vi "think_and_act.vi"(8 "error in (no error)":errorcluster, 9 "antState":T1, 10 "pieceOfWorld":T4[][](array[typedef]), 11 "Igor in":refnum<class "PolyVIEW.lvclass">) -> (0 "error out":errorcluster, 2 "action":T2, 3 "Igor out":refnum<class "PolyVIEW.lvclass">)   [LabVIEW 2015, in "PolyVIEW.lvclass"]
doc: "Ant thinks and chooses action\nCreated by Artem Shevelev\nshevelev.pro\nartem@shevelev.pro\nLabVIEW Portal: https://labviewportal.org/memberlist.php?mode=viewprofile&u=2340"
uses:
  PolyVIEW.lvclass
  actors/world/typedefs/worldCell_cluster.ctl
  actors/world/typedefs/markValue_cluster.ctl
  actors/world/typedefs/markValue.ctl
  actors/world/typedefs/markVolume.ctl
  actors/world/typedefs/amountOfFood.ctl
  actors/world/typedefs/anthillType_enum.ctl
  ant_base/action_cluster.ctl
  ant_base/actionType_enum.ctl
  ant_base/antState_cluster.ctl
  ant_base/ant_base.lvclass/ant_base.ctl
  Admin memo.ctl
  ant_base/memory_limit_const.vi
  move_forvard.vi
  move_back.vi
  ant_base/ant_base.lvclass
  actors/world/world.lvlib
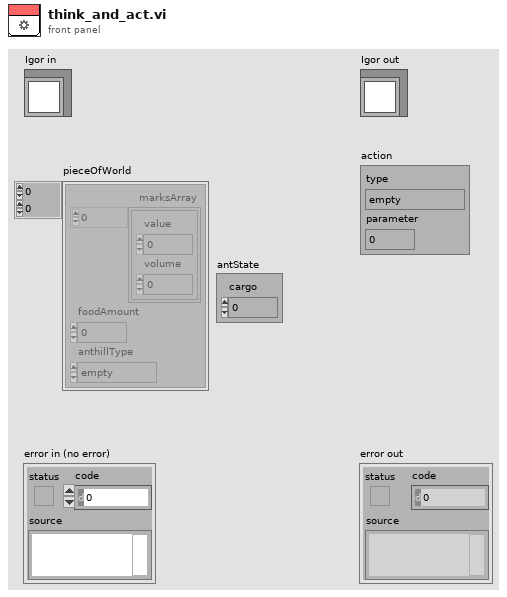
[diagram p1: front panel]
types:
  T1 = typedef "ant_base.lvclass/antState_cluster.ctl" = cluster{"cargo":u8}
  T2 = typedef "ant_base.lvclass/action_cluster.ctl" = cluster{"type":T3, "parameter":dbl}
  T3 = typedef "ant_base.lvclass/actionType_enum.ctl" = enum8{"empty", "move", "take", "put", "mark"}
  T4 = typedef "world.lvlib/worldCell_cluster.ctl" = cluster{"marksArray":T5[], "foodAmount":T8, "anthillType":T9}
  T5 = typedef "world.lvlib/markValue_cluster.ctl" = cluster{"value":T6, "volume":T7}
  T6 = typedef "world.lvlib/markValue.ctl" = u8
  T7 = typedef "world.lvlib/markVolume.ctl" = u16
  T8 = typedef "world.lvlib/amountOfFood.ctl" = i32
  T9 = typedef "world.lvlib/anthillType_enum.ctl" = enum16{"empty", "own", "rival"}
  T10 = typedef "PolyVIEW.lvclass/Admin memo.ctl" = cluster{"role":i32, "max vol":i32, "vol step":i32, "num of az":i32, "mode mark":i32, "arr of blk":i32[], "arr of az":i32[]}
  T11 = typedef "PolyVIEW.lvclass/Memory.ctl" = cluster{"role":i32, "az":i32, "blk az":i32, "steps I":u32, "add rad":i32, "steps II":u32, "mode mark":u32, "base az":u32, "num of az":u32, "mark 253":u32, "mode":u32, "commands":i32[]}
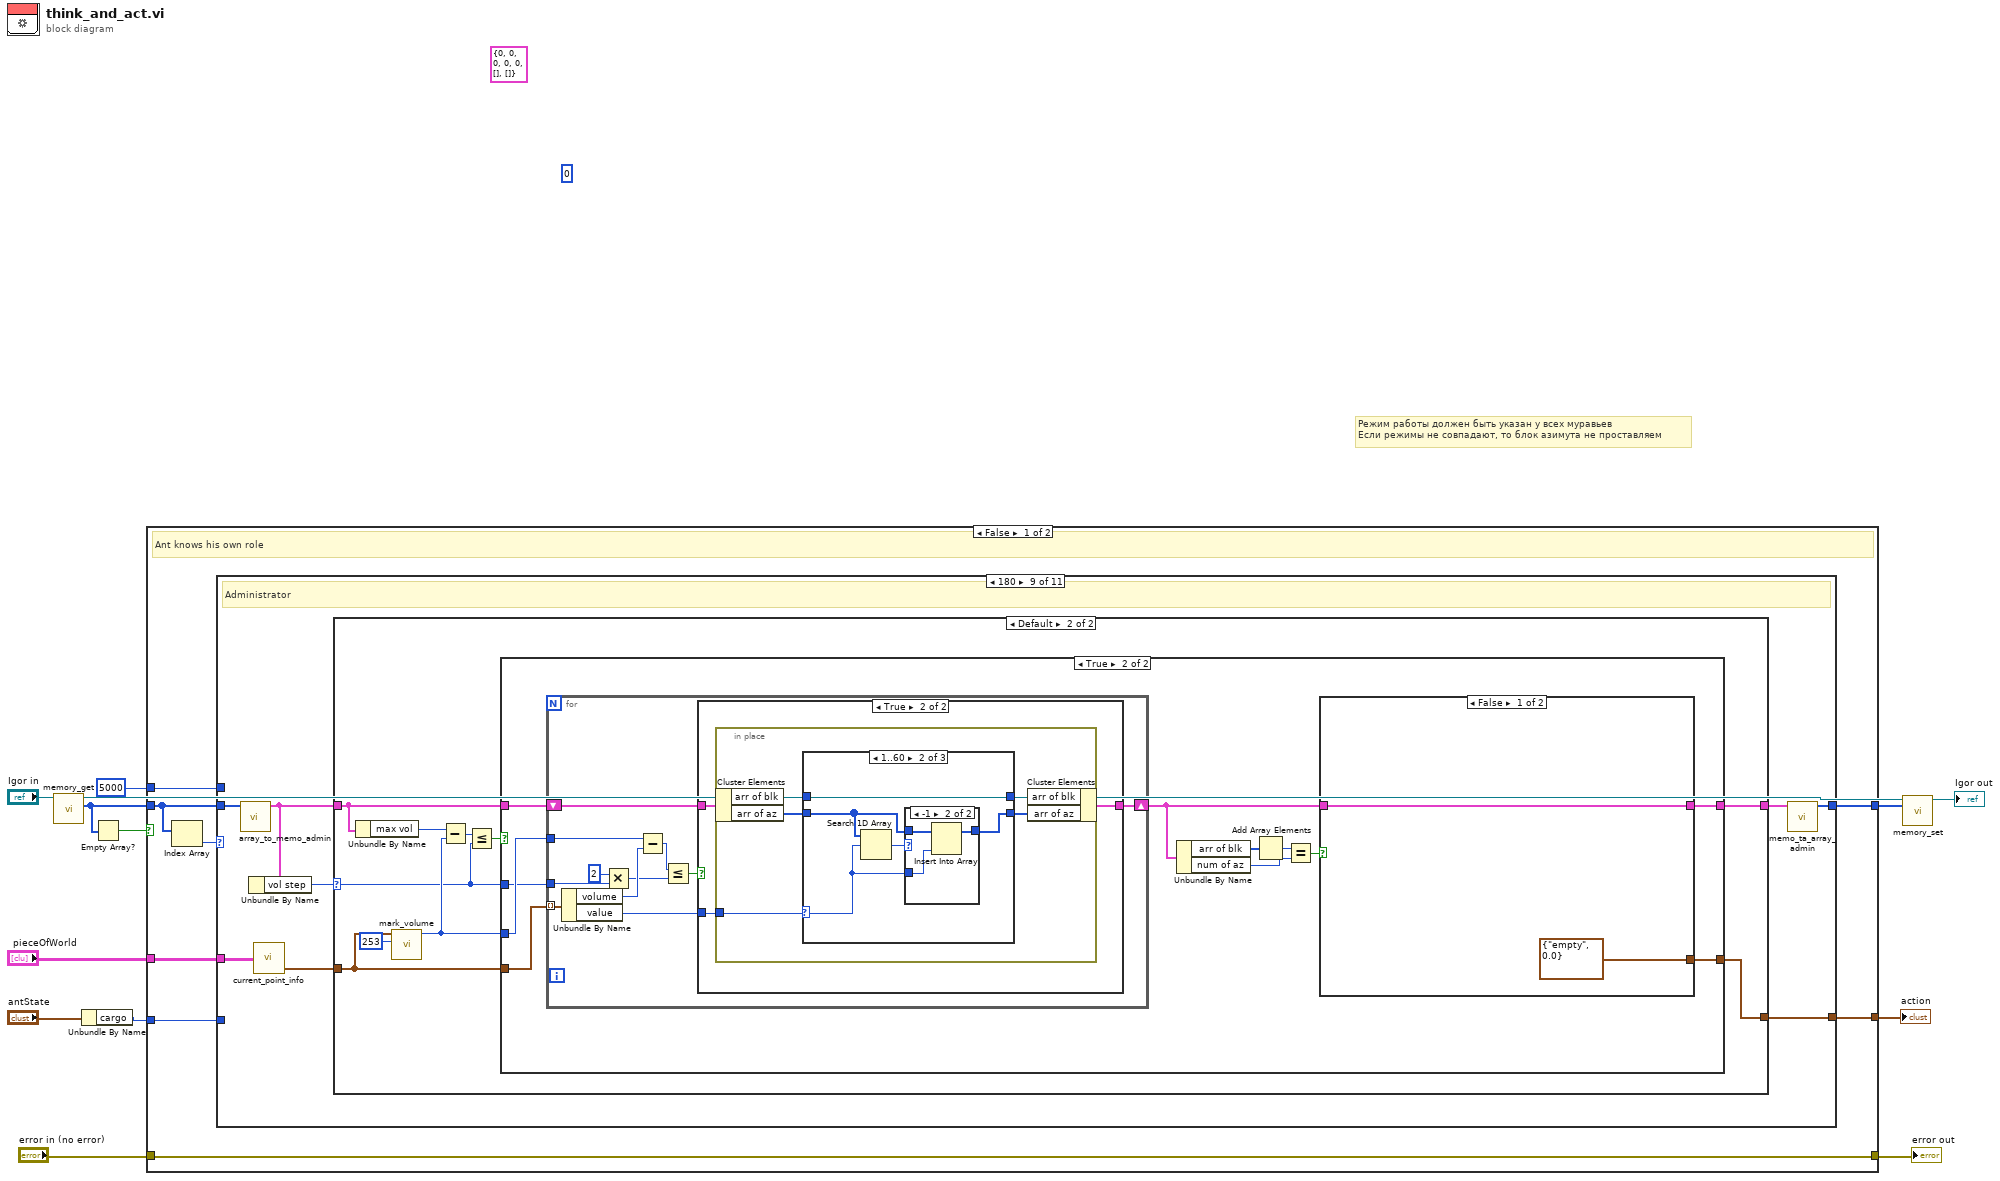
[diagram p0: block diagram]
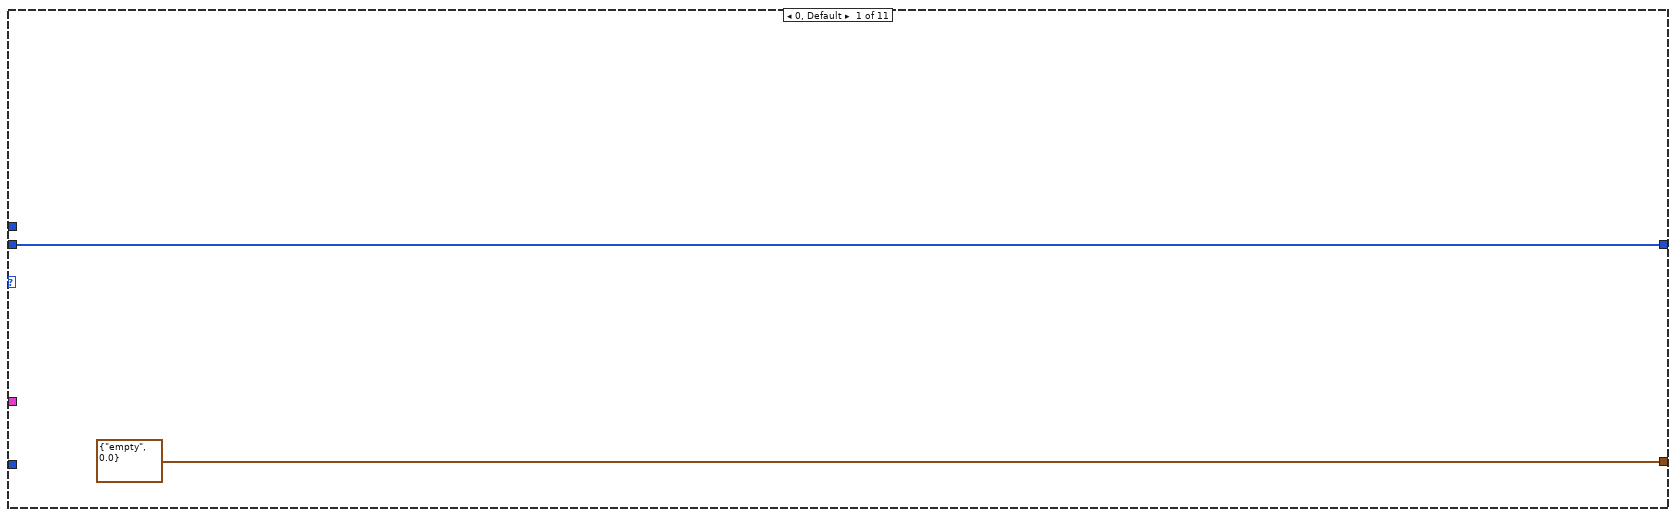
[diagram p2: hidden frame]
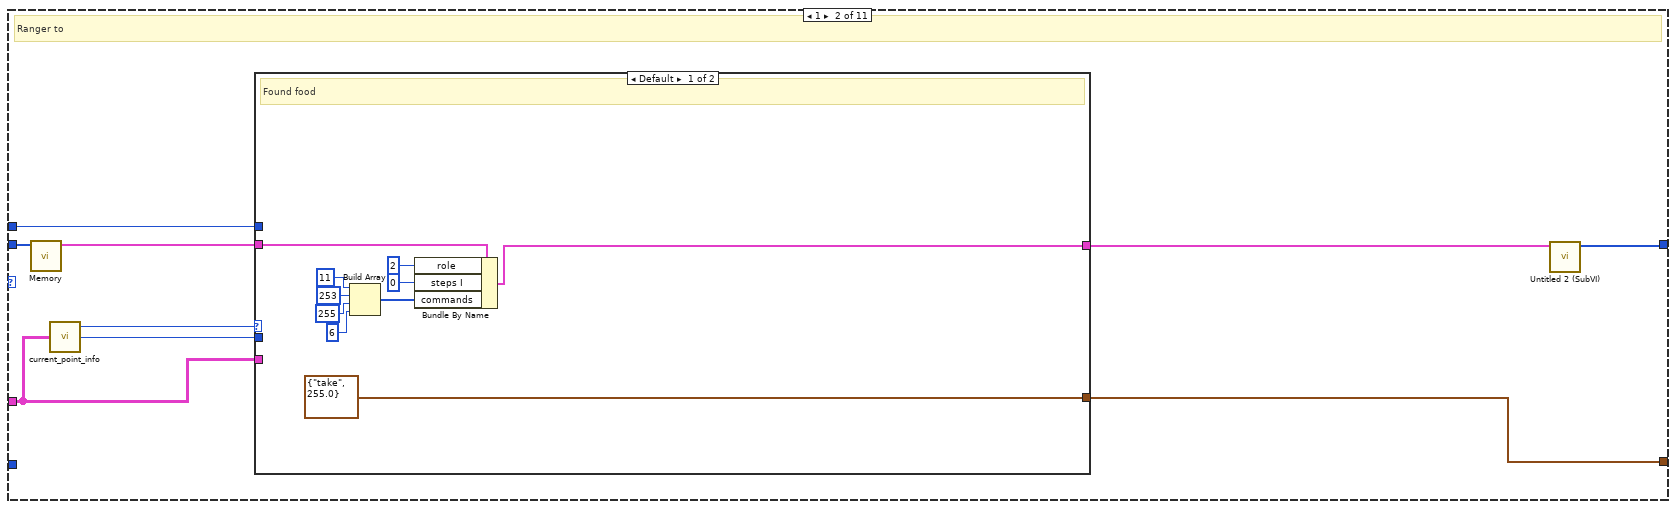
[diagram p3: hidden frame]
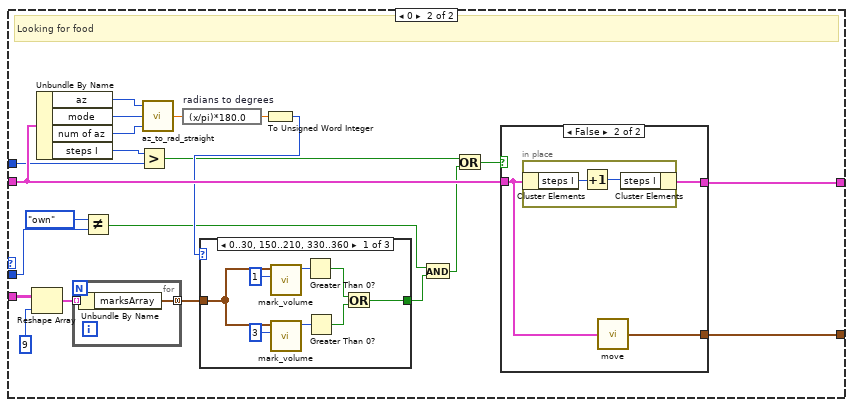
[diagram p4: hidden frame]
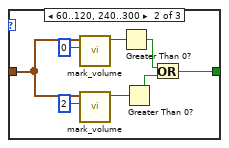
[diagram p5: hidden frame]
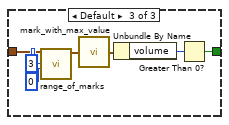
[diagram p6: hidden frame]
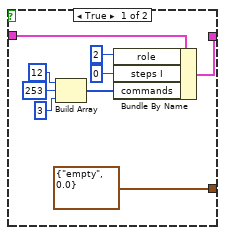
[diagram p7: hidden frame]
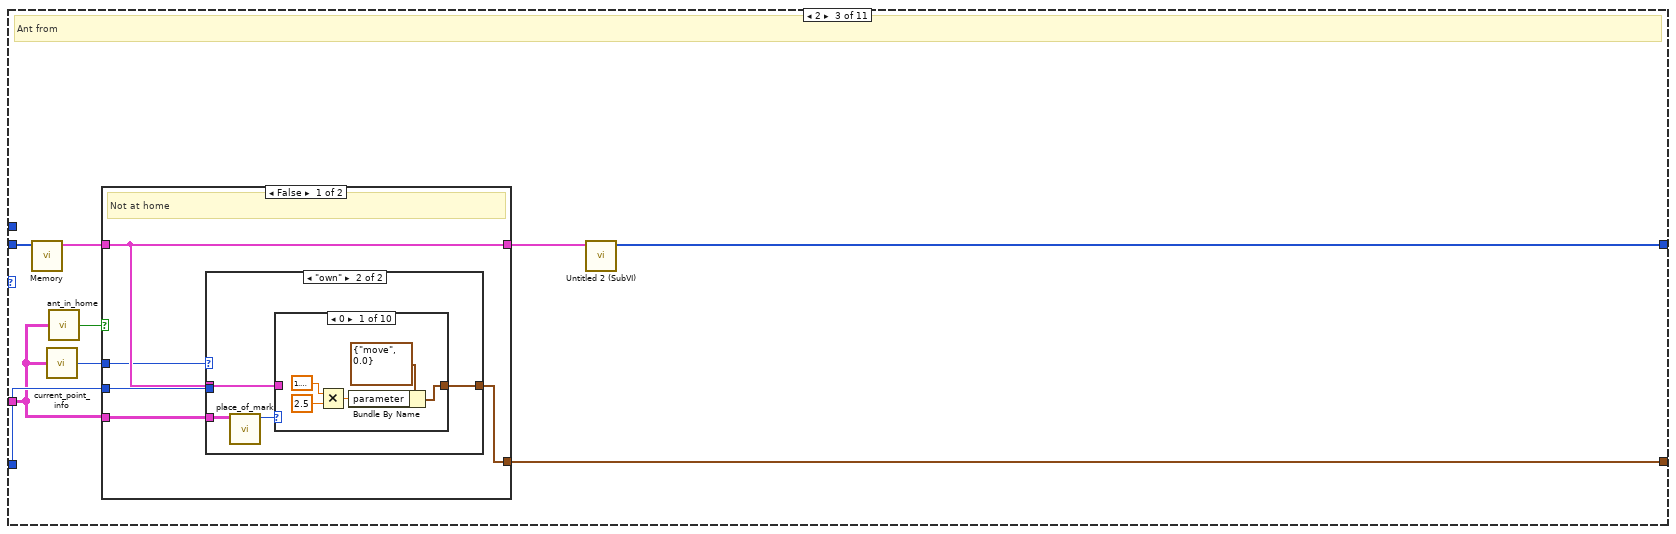
[diagram p8: hidden frame]
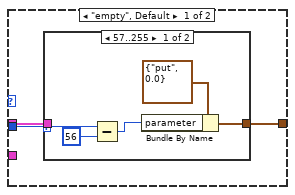
[diagram p9: hidden frame]
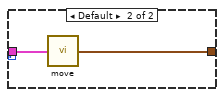
[diagram p10: hidden frame]
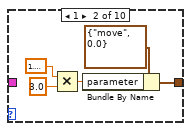
[diagram p11: hidden frame]
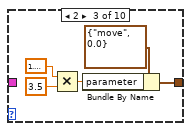
[diagram p12: hidden frame]
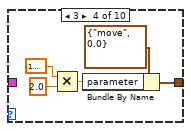
[diagram p13: hidden frame]
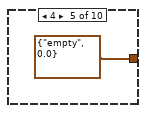
[diagram p14: hidden frame]
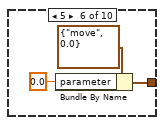
[diagram p15: hidden frame]
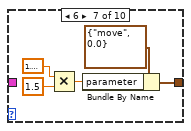
[diagram p16: hidden frame]
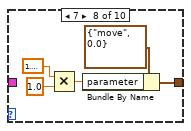
[diagram p17: hidden frame]
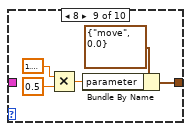
[diagram p18: hidden frame]
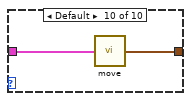
[diagram p19: hidden frame]
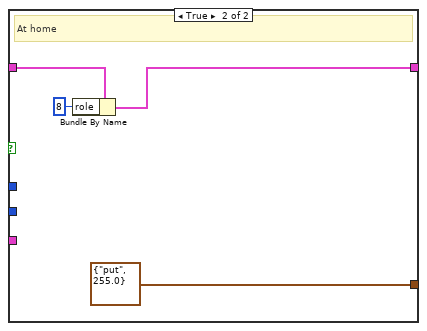
[diagram p20: hidden frame]
diagram:
  (unwired) T6 0 ("value")
  (unwired) T10 {"role"=0, "max vol"=0, "vol step"=0, "num of az"=0, "mode mark"=0, "arr of blk"=[], "arr of az"=[]}
  # "Режим работы должен быть указан у всех муравьев\nЕсли режимы не совпадают, то блок азимута не проставляем"
  n1 = call "memory_get.vi"("ant_base in"="Igor in") -> ("memory"=w3:u8[], "ant_base out"=w8:refnum<class "PolyVIEW.lvclass">)  [unwired: 8 in, 1 out]
  n2 = Unbundle By Name("antState") -> ("cargo"=w4:u8)
  n3 = Empty Array?(array=w3) -> (empty?=w10:bool)
  n4 = case shown="False" w10 {
    tunnel: [w14 w737] -> w5
    tunnel: [w20 w736] -> w13
    tunnel: "error in (no error)" -> [w14 w737]
    tunnel: w3 -> [w19 w733]
    tunnel: "pieceOfWorld" -> [w18 w732]
    tunnel: [w17 w734] -> w7
    tunnel: w4 -> [w16 _]
    tunnel: u32 5000 ("y") -> [w15 _]
    frame False {
      # "Ant knows his own role"
      n5 = Index Array(array=w19) -> (element=w21:u8)  [unwired: 1 in]
      n6 = case shown="180" w21 {
        tunnel: [T2 {"type"=enum."empty", "parameter"=0.0} ("action") w32 w112 T2 {"type"=enum."empty", "parameter"=0.0} ("action") w244 w321 w402 w462 w586 T2 {"type"=enum."mark", "parameter"=254.0} ("action") T2 {"type"=enum."empty", "parameter"=0.0} ("action")] -> w20
        tunnel: w19 -> [w22 w30 w110 w191 w242 w319 w404 w463 w583 w723 w728]
        tunnel: w18 -> [_ w31 w104 w182 w243 w320 w392 w459 w585 _ _]
        tunnel: [w22 w27 w107 w189 w239 w316 w403 w461 w579 w722 w727] -> w17
        tunnel: w16 -> [_ _ w106 _ _ _ _ _ _ _ _]
        tunnel: w15 -> [_ w26 _ _ w236 w313 _ _ _ _ _]
        frame 0, Default {
        }
        frame 1 {
          # "Ranger to"
          n7 = call "Memory.vi"("memory"=w30) -> ("output cluster"=w29:T11)  [unwired: 10 in]
          n8 = call "current_point_info.vi"("pieceOfWorld"=w31) -> ("foodAmount"=w25:T8, "anthillType"=w24:T9)  [unwired: 1 out]
          n9 = case shown="Default" w25 {
            tunnel: [T2 {"type"=enum."take", "parameter"=255.0} ("action") w64] -> w32
            tunnel: w29 -> [w40 w58]
            tunnel: [w39 w63] -> w28
            tunnel: w31 -> [_ w60]
            tunnel: w24 -> [_ w52]
            tunnel: w26 -> [_ w45]
            frame Default {
              # "Found food"
              n10 = Build Array(11 ("element"), 253 ("element"), 255 ("element"), 6 ("element")) -> (w35:i32[])
              n11 = Bundle By Name(cluster=w40, "role"=u8 2 ("new element/subarray"), "steps I"=u32 0 ("Steps I"), "commands"=w35) -> (w39:T11)
            }
            frame 0 {
              # "Looking for food"
              n12 = Reshape Array(w60, 9 ("dimension size")) -> (w61:T4[])
              n13 = Unbundle By Name(w58) -> ("az"=w43:i32, "mode"=w44:u32, "num of az"=w57:u32, "steps I"=w49:u32)
              n14 = for {
                tunnel: w61 -> [w89] mode=indexing
                tunnel: [w88] -> w59 mode=concatenating
                n15 = Unbundle By Name(w89) -> ("marksArray"=w88:T5[])
              }
              n16 = Not Equal?(x=anthillType_enum."own", y=w52) -> (x != y?=w50:bool)
              n17 = Greater?(x=w49, y=w45) -> (0:w48:bool)
              n18 = call "az_to_rad_straight.vi"("az quantity"=w57, "mode"=w44, "az"=w43) -> ("rad"=w56:dbl)
              n19 = expression code="(x/pi)*180.0" "radians to degrees"(w56) -> (w55:dbl)
              n20 = To Unsigned Word Integer(number=w55) -> (unsigned 16bit integer=w54:u16)
              n21 = case shown="0..30, 150..210, 330..360" w54 {
                tunnel: w59 -> [w72 w80 w85]
                tunnel: [w65 w73 w81] -> w53
                frame 0..30, 150..210, 330..360 {
                  n22 = call "mark_volume.vi"("element"=T6 1, "marksArray"=w72) -> ("volume"=w68:T7)  [unwired: 9 in]
                  n23 = call "mark_volume.vi"("element"=T6 3, "marksArray"=w72) -> ("volume"=w69:T7)  [unwired: 9 in]
                  n24 = Greater Than 0?(x=w68) -> (x > 0?=w66:bool)
                  n25 = Greater Than 0?(x=w69) -> (x > 0?=w67:bool)
                  n26 = Or(x=w66, y=w67) -> (x .or. y?=w65:bool)
                }
                frame 60..120, 240..300 {
                  n27 = call "mark_volume.vi"("element"=T6 0, "marksArray"=w80) -> ("volume"=w76:T7)  [unwired: 9 in]
                  n28 = call "mark_volume.vi"("element"=T6 2, "marksArray"=w80) -> ("volume"=w77:T7)  [unwired: 9 in]
                  n29 = Greater Than 0?(x=w76) -> (x > 0?=w74:bool)
                  n30 = Greater Than 0?(x=w77) -> (x > 0?=w75:bool)
                  n31 = Or(x=w74, y=w75) -> (x .or. y?=w73:bool)
                }
                frame Default {
                  n32 = call "range_of_marks.vi"("lower limit"=T6 0, "upper limit"=T6 3, "marksArray"=w85) -> ("Array"=w84:T5[])  [unwired: 8 in]
                  n33 = call "mark_with_max_value.vi"("marksArray"=w84) -> ("markValue"=w83:T5)
                  n34 = Unbundle By Name(w83) -> ("volume"=w82:T7)
                  n35 = Greater Than 0?(x=w82) -> (x > 0?=w81:bool)
                }
              }
              n36 = And(x=w50, y=w53) -> (x .and. y?=w47:bool)
              n37 = Or(x=w48, y=w47) -> (x .or. y?=w46:bool)
              n38 = case shown="False" w46 {
                tunnel: [T2 {"type"=enum."empty", "parameter"=0.0} ("action") w101] -> w64
                tunnel: w58 -> [w95 w100]
                tunnel: [w96 w99] -> w63
                frame True {
                  n39 = Build Array(12 ("element"), 253 ("element"), 3 ("element")) -> (w91:i32[])
                  n40 = Bundle By Name(cluster=w95, "role"=u8 2 ("new element/subarray"), "steps I"=u32 0 ("Steps I"), "commands"=w91) -> (w96:T11)
                }
                frame False {
                  n41 = in-place {
                    n42 = in-place-cluster #1(w100) -> ("steps I"=w103:u32)
                    n43 = Increment(x=w103) -> (x+1=w102:u32)
                    n44 = in-place-cluster #1("steps I"=w102) -> (w99:T11)
                  }
                  n45 = call-poly "move.vi"("output cluster"=w100) -> ("action"=w101:T2)
                }
              }
            }
          }
          n46 = call "Untitled 2 (SubVI).vi"(11:w28) -> ("appended array"=w27:u32[])  [unwired: 10 in]
        }
        frame 2 {
          # "Ant from"
          n47 = call "Memory.vi"("memory"=w110) -> ("output cluster"=w109:T11)  [unwired: 10 in]
          n48 = call "current_point_info.vi"("pieceOfWorld"=w104) -> ("anthillType"=w105:T9)  [unwired: 2 out]
          n49 = call "ant_in_home.vi"("pieceOfWorld"=w104) -> ("x .and. y?"=w111:bool)
          n50 = case shown="False" w111 {
            tunnel: [w116 T2 {"type"=enum."put", "parameter"=255.0} ("action")] -> w112
            tunnel: w109 -> [w117 w176]
            tunnel: [w117 w173] -> w108
            tunnel: w106 -> [w115 _]
            tunnel: w105 -> [w114 _]
            tunnel: w104 -> [w113 _]
            frame False {
              # "Not at home"
              n51 = case shown="\"own\"" w114 {
                tunnel: w117 -> [w120 w130]
                tunnel: [w119 w129] -> w116
                tunnel: w115 -> [w118 _]
                tunnel: w113 -> [_ w128]
                frame "empty", Default {
                  n52 = case shown="57..255" w118 {
                    selector: w118 -> [w124 _]
                    tunnel: w120 -> [_ w127]
                    tunnel: [w121 w126] -> w119
                    frame 57..255 {
                      n53 = Subtract(x=w124, y=u8 56) -> (x-y=w122:u8)
                      n54 = Bundle By Name(cluster=T2 {"type"=enum."put", "parameter"=0.0} ("action"), "parameter"=w122) -> (w121:T2)
                    }
                    frame Default {
                      n55 = call-poly "move.vi"("output cluster"=w127) -> ("action"=w126:T2)
                    }
                  }
                }
                frame "own" {
                  n56 = call "place_of_mark.vi"("pieceOfWorld in"=w128) -> ("f"=w131:i32)  [unwired: 10 in]
                  n57 = case shown="0" w131 {
                    tunnel: w130 -> [_ _ _ _ _ _ _ _ _ w172]
                    tunnel: [w136 w141 w146 w151 T2 {"type"=enum."empty", "parameter"=0.0} ("action") w155 w160 w165 w170 w171] -> w129
                    frame 0 {
                      n58 = Multiply(x=1.5707963267948966, y=2.5) -> (x*y=w132:dbl)
                      n59 = Bundle By Name(cluster=T2 {"type"=enum."move", "parameter"=0.0} ("action"), "parameter"=w132) -> (w136:T2)
                    }
                    frame 1 {
                      n60 = Multiply(x=1.5707963267948966, y=3.0) -> (x*y=w137:dbl)
                      n61 = Bundle By Name(cluster=T2 {"type"=enum."move", "parameter"=0.0} ("action"), "parameter"=w137) -> (w141:T2)
                    }
                    frame 2 {
                      n62 = Multiply(x=1.5707963267948966, y=3.5) -> (x*y=w142:dbl)
                      n63 = Bundle By Name(cluster=T2 {"type"=enum."move", "parameter"=0.0} ("action"), "parameter"=w142) -> (w146:T2)
                    }
                    frame 3 {
                      n64 = Multiply(x=1.5707963267948966, y=2.0) -> (x*y=w147:dbl)
                      n65 = Bundle By Name(cluster=T2 {"type"=enum."move", "parameter"=0.0} ("action"), "parameter"=w147) -> (w151:T2)
                    }
                    frame 4 {
                    }
                    frame 5 {
                      n66 = Bundle By Name(cluster=T2 {"type"=enum."move", "parameter"=0.0} ("action"), "parameter"=0.0) -> (w155:T2)
                    }
                    frame 6 {
                      n67 = Multiply(x=1.5707963267948966, y=1.5) -> (x*y=w156:dbl)
                      n68 = Bundle By Name(cluster=T2 {"type"=enum."move", "parameter"=0.0} ("action"), "parameter"=w156) -> (w160:T2)
                    }
                    frame 7 {
                      n69 = Multiply(x=1.5707963267948966, y=1.0) -> (x*y=w161:dbl)
                      n70 = Bundle By Name(cluster=T2 {"type"=enum."move", "parameter"=0.0} ("action"), "parameter"=w161) -> (w165:T2)
                    }
                    frame 8 {
                      n71 = Multiply(x=1.5707963267948966, y=0.5) -> (x*y=w166:dbl)
                      n72 = Bundle By Name(cluster=T2 {"type"=enum."move", "parameter"=0.0} ("action"), "parameter"=w166) -> (w170:T2)
                    }
                    frame Default {
                      n73 = call-poly "move.vi"("output cluster"=w172) -> ("action"=w171:T2)
                    }
                  }
                }
              }
            }
            frame True {
              # "At home"
              n74 = Bundle By Name(cluster=w176, "role"=u8 8 ("y")) -> (w173:T11)
            }
          }
          n75 = call "Untitled 2 (SubVI).vi"(11:w108) -> ("appended array"=w107:u32[])  [unwired: 10 in]
        }
        frame 3 {
          # "Ant-on-duty"
          n76 = call "Memory.vi"("memory"=w191) -> ("output cluster"=w180:T11)  [unwired: 10 in]
          n77 = call "current_point_info.vi"("pieceOfWorld"=w182) -> ("marksArray"=w179:T5[])  [unwired: 2 out]
          n78 = call "range_of_marks.vi"("lower limit"=T6 251, "upper limit"=T6 252, "marksArray"=w179) -> ("Array"=w186:T5[])  [unwired: 8 in]
          n79 = call "mark_with_max_volume.vi"("marksArray"=w186) -> ("markValue"=w185:T5)
          n80 = Unbundle By Name(w180) -> ("mode mark"=w178:u32)
          n81 = Unbundle By Name(w185) -> ("value"=w177:T6)
          n82 = Equal To 0?(x=w177) -> (x = 0?=w183:bool)
          n83 = Equal?(x=w178, y=w177) -> (x = y?=w184:bool)
          n84 = Or(x=w184, y=w183) -> (x .or. y?=w181:bool)
          n85 = case shown="True" w181 {
            tunnel: [w197 w223] -> w190
            tunnel: w180 -> [w196 w222]
            tunnel: w179 -> [_ w216]
            tunnel: w177 -> [w193 _]
            frame False {
              n86 = Unbundle By Name(w196) -> ("base az"=w194:u32, "mode"=w195:u32)
              n87 = case shown="Default" w194 {
                selector: w194 -> [w199 _]
                tunnel: [w202 w210] -> w197
                tunnel: w196 -> [w203 w209]
                tunnel: w195 -> [w201 w207]
                tunnel: w193 -> [w198 w205]
                frame Default {
                  n88 = Increment(x=w201) -> (x+1=w200:u32)
                  n89 = Bundle By Name(cluster=w203, "role"=1, "az"=w199, "mode"=w200, "mode mark"=w198) -> (w202:T11)
                }
                frame 0 {
                  n90 = Increment(x=w207) -> (x+1=w206:u32)
                  n91 = Bundle By Name(cluster=w209, "role"=3, "mode"=w206, "mode mark"=w205) -> (w210:T11)
                }
              }
            }
            frame True {
              n92 = call "range_of_marks.vi"("lower limit"=T6 121, "upper limit"=T6 180, "marksArray"=w216) -> ("Array"=w218:T5[])  [unwired: 8 in]
              n93 = call "range_of_marks.vi"("lower limit"=T6 254, "upper limit"=T6 255, "marksArray"=w216) -> ("Array"=w212:T5[])  [unwired: 8 in]
              n94 = call "mark_with_max_volume.vi"("marksArray"=w218) -> ("markValue"=w219:T5)
              n95 = call "mark_with_max_volume.vi"("marksArray"=w212) -> ("markValue"=w213:T5)
              n96 = Unbundle By Name(w219) -> ("value"=w217:T6)
              n97 = Unbundle By Name(w213) -> ("value"=w211:T6)
              n98 = case shown="255" w211 {
                tunnel: [w224 w227] -> w223
                tunnel: w222 -> [w224 w226]
                tunnel: w217 -> [_ w225]
                frame 254, Default {
                }
                frame 255 {
                  n99 = case shown="121..180" w225 {
                    selector: w225 -> [w233 _]
                    tunnel: w226 -> [w230 w235]
                    tunnel: [w234 w235] -> w227
                    frame 121..180 {
                      # "Got a target"
                      n100 = Subtract(x=w233, y=T6 120) -> (x-y=w231:T6)
                      n101 = Bundle By Name(cluster=w230, "role"=4 ("Role"), "az"=w231, "steps I"=u32 0 ("Steps I")) -> (w234:T11)
                    }
                    frame Default {
                      # "Expecting a target"
                    }
                  }
                }
              }
            }
          }
          n102 = call "Untitled 2 (SubVI).vi"(11:w190) -> ("appended array"=w189:u32[])  [unwired: 10 in]
        }
        frame 4 {
          # "Worker to"
          n103 = call "Memory.vi"("memory"=w242) -> ("output cluster"=w241:T11)  [unwired: 10 in]
          n104 = call "current_point_info.vi"("pieceOfWorld"=w243) -> ("foodAmount"=w238:T8, "anthillType"=w237:T9)  [unwired: 1 out]
          n105 = case shown="0" w238 {
            tunnel: [T2 {"type"=enum."take", "parameter"=255.0} ("action") w273] -> w244
            tunnel: w241 -> [w250 w267]
            tunnel: [w249 w272] -> w240
            tunnel: w243 -> [_ w269]
            tunnel: w237 -> [_ w259]
            tunnel: w236 -> [_ w256]
            frame Default {
              # "Found food"
              n106 = Build Array(255 ("element"), 3 ("element")) -> (w247:i32[])
              n107 = Bundle By Name(cluster=w250, "role"=u8 2 ("new element/subarray"), "steps I"=u32 0 ("Steps I"), "commands"=w247) -> (w249:T11)
            }
            frame 0 {
              # "Looking for food"
              n108 = Reshape Array(w269, 9 ("dimension size")) -> (w270:T4[])
              n109 = Unbundle By Name(w267) -> ("az"=w266:i32, "num of az"=w265:u32, "steps I"=w257:u32)
              n110 = for {
                tunnel: w270 -> [w298] mode=indexing
                tunnel: [w297] -> w268 mode=concatenating
                n111 = Unbundle By Name(w298) -> ("marksArray"=w297:T5[])
              }
              n112 = Not Equal?(x=anthillType_enum."own", y=w259) -> (x != y?=w258:bool)
              n113 = Greater?(x=w257, y=w256) -> (0:w253:bool)
              n114 = call "az_to_rad_straight.vi"("az quantity"=w265, "az"=w266) -> ("rad"=w264:dbl)  [unwired: 1 in]
              n115 = expression code="(x/pi)*180.0" "radians to degrees"(w264) -> (w263:dbl)
              n116 = To Unsigned Word Integer(number=w263) -> (unsigned 16bit integer=w262:u16)
              n117 = case shown="60..120, 240..300" w262 {
                tunnel: w268 -> [w281 w289 w294]
                tunnel: [w274 w282 w290] -> w261
                frame 0..30, 150..210, 330..360 {
                  n118 = call "mark_volume.vi"("element"=T6 1, "marksArray"=w281) -> ("volume"=w277:T7)  [unwired: 9 in]
                  n119 = call "mark_volume.vi"("element"=T6 3, "marksArray"=w281) -> ("volume"=w278:T7)  [unwired: 9 in]
                  n120 = Greater Than 0?(x=w277) -> (x > 0?=w275:bool)
                  n121 = Greater Than 0?(x=w278) -> (x > 0?=w276:bool)
                  n122 = Or(x=w275, y=w276) -> (x .or. y?=w274:bool)
                }
                frame 60..120, 240..300 {
                  n123 = call "mark_volume.vi"("element"=T6 0, "marksArray"=w289) -> ("volume"=w285:T7)  [unwired: 9 in]
                  n124 = call "mark_volume.vi"("element"=T6 2, "marksArray"=w289) -> ("volume"=w286:T7)  [unwired: 9 in]
                  n125 = Greater Than 0?(x=w285) -> (x > 0?=w283:bool)
                  n126 = Greater Than 0?(x=w286) -> (x > 0?=w284:bool)
                  n127 = Or(x=w283, y=w284) -> (x .or. y?=w282:bool)
                }
                frame Default {
                  n128 = call "range_of_marks.vi"("lower limit"=T6 0, "upper limit"=T6 3, "marksArray"=w294) -> ("Array"=w293:T5[])  [unwired: 8 in]
                  n129 = call "mark_with_max_value.vi"("marksArray"=w293) -> ("markValue"=w292:T5)
                  n130 = Unbundle By Name(w292) -> ("volume"=w291:T7)
                  n131 = Greater Than 0?(x=w291) -> (x > 0?=w290:bool)
                }
              }
              n132 = And(x=w258, y=w261) -> (x .and. y?=w255:bool)
              n133 = Or(x=w253, y=w255) -> (x .or. y?=w254:bool)
              n134 = case shown="True" w254 {
                tunnel: [T2 {"type"=enum."empty", "parameter"=0.0} ("action") w310] -> w273
                tunnel: w267 -> [w303 w309]
                tunnel: [w304 w308] -> w272
                frame True {
                  n135 = Build Array(12 ("element"), 253 ("element"), 3 ("element")) -> (w299:i32[])
                  n136 = Bundle By Name(cluster=w303, "role"=u8 2 ("new element/subarray"), "steps I"=u8 0 ("new element/subarray"), "commands"=w299) -> (w304:T11)
                }
                frame False {
                  n137 = in-place {
                    n138 = in-place-cluster #2(w309) -> ("steps I"=w312:u32)
                    n139 = Increment(x=w312) -> (x+1=w311:u32)
                    n140 = in-place-cluster #2("steps I"=w311) -> (w308:T11)
                  }
                  n141 = call-poly "move.vi"("output cluster"=w309) -> ("action"=w310:T2)
                }
              }
            }
          }
          n142 = call "Untitled 2 (SubVI).vi"(11:w240) -> ("appended array"=w239:u32[])  [unwired: 10 in]
        }
        frame 6 {
          # "Provider to"
          n143 = call "Memory.vi"("memory"=w319) -> ("output cluster"=w318:T11)  [unwired: 10 in]
          n144 = call "current_point_info.vi"("pieceOfWorld"=w320) -> ("foodAmount"=w315:T8, "anthillType"=w314:T9)  [unwired: 1 out]
          n145 = case shown="0" w315 {
            tunnel: [T2 {"type"=enum."take", "parameter"=255.0} ("action") w350] -> w321
            tunnel: w318 -> [w327 w344]
            tunnel: [w326 w349] -> w317
            tunnel: w320 -> [_ w346]
            tunnel: w314 -> [_ w336]
            tunnel: w313 -> [_ w333]
            frame Default {
              # "Found food"
              n146 = Build Array(255 ("element"), 6 ("element")) -> (w324:i32[])
              n147 = Bundle By Name(cluster=w327, "role"=u8 2 ("new element/subarray"), "steps I"=u32 0 ("Steps I"), "commands"=w324) -> (w326:T11)
            }
            frame 0 {
              # "Looking for food"
              n148 = Reshape Array(w346, 9 ("dimension size")) -> (w347:T4[])
              n149 = Unbundle By Name(w344) -> ("az"=w343:i32, "num of az"=w342:u32, "steps I"=w334:u32)
              n150 = for {
                tunnel: w347 -> [w375] mode=indexing
                tunnel: [w374] -> w345 mode=concatenating
                n151 = Unbundle By Name(w375) -> ("marksArray"=w374:T5[])
              }
              n152 = Not Equal?(x=anthillType_enum."own", y=w336) -> (x != y?=w335:bool)
              n153 = Greater?(x=w334, y=w333) -> (0:w330:bool)
              n154 = call "az_to_rad_straight.vi"("az quantity"=w342, "az"=w343) -> ("rad"=w341:dbl)  [unwired: 1 in]
              n155 = expression code="(x/pi)*180.0" "radians to degrees"(w341) -> (w340:dbl)
              n156 = To Unsigned Word Integer(number=w340) -> (unsigned 16bit integer=w339:u16)
              n157 = case shown="0..30, 150..210, 330..360" w339 {
                tunnel: w345 -> [w358 w366 w371]
                tunnel: [w351 w359 w367] -> w338
                frame 0..30, 150..210, 330..360 {
                  n158 = call "mark_volume.vi"("element"=T6 1, "marksArray"=w358) -> ("volume"=w354:T7)  [unwired: 9 in]
                  n159 = call "mark_volume.vi"("element"=T6 3, "marksArray"=w358) -> ("volume"=w355:T7)  [unwired: 9 in]
                  n160 = Greater Than 0?(x=w354) -> (x > 0?=w352:bool)
                  n161 = Greater Than 0?(x=w355) -> (x > 0?=w353:bool)
                  n162 = Or(x=w352, y=w353) -> (x .or. y?=w351:bool)
                }
                frame 60..120, 240..300 {
                  n163 = call "mark_volume.vi"("element"=T6 0, "marksArray"=w366) -> ("volume"=w362:T7)  [unwired: 9 in]
                  n164 = call "mark_volume.vi"("element"=T6 2, "marksArray"=w366) -> ("volume"=w363:T7)  [unwired: 9 in]
                  n165 = Greater Than 0?(x=w362) -> (x > 0?=w360:bool)
                  n166 = Greater Than 0?(x=w363) -> (x > 0?=w361:bool)
                  n167 = Or(x=w360, y=w361) -> (x .or. y?=w359:bool)
                }
                frame Default {
                  n168 = call "range_of_marks.vi"("lower limit"=T6 0, "upper limit"=T6 3, "marksArray"=w371) -> ("Array"=w370:T5[])  [unwired: 8 in]
                  n169 = call "mark_with_max_value.vi"("marksArray"=w370) -> ("markValue"=w369:T5)
                  n170 = Unbundle By Name(w369) -> ("volume"=w368:T7)
                  n171 = Greater Than 0?(x=w368) -> (x > 0?=w367:bool)
                }
              }
              n172 = And(x=w335, y=w338) -> (x .and. y?=w332:bool)
              n173 = Or(x=w330, y=w332) -> (x .or. y?=w331:bool)
              n174 = case shown="True" w331 {
                tunnel: [T2 {"type"=enum."empty", "parameter"=0.0} ("action") w387] -> w350
                tunnel: w344 -> [w380 w386]
                tunnel: [w381 w385] -> w349
                frame True {
                  n175 = Build Array(12 ("element"), 253 ("element"), 3 ("element")) -> (w376:i32[])
                  n176 = Bundle By Name(cluster=w380, "role"=u8 2 ("new element/subarray"), "steps I"=u8 0 ("new element/subarray"), "commands"=w376) -> (w381:T11)
                }
                frame False {
                  n177 = in-place {
                    n178 = in-place-cluster #3(w386) -> ("steps I"=w389:u32)
                    n179 = Increment(x=w389) -> (x+1=w388:u32)
                    n180 = in-place-cluster #3("steps I"=w388) -> (w385:T11)
                  }
                  n181 = call-poly "move.vi"("output cluster"=w386) -> ("action"=w387:T2)
                }
              }
            }
          }
          n182 = call "Untitled 2 (SubVI).vi"(11:w317) -> ("appended array"=w316:u32[])  [unwired: 10 in]
        }
        frame 8 {
          n183 = call "Memory.vi"("memory"=w404) -> ("output cluster"=w391:T11)  [unwired: 10 in]
          n184 = call "current_point_info.vi"("pieceOfWorld"=w392) -> ("marksArray"=w393:T5[])  [unwired: 2 out]
          n185 = Unbundle By Name(w391) -> ("mode mark"=w397:u32)
          n186 = call "range_of_marks.vi"("lower limit"=T6 251, "upper limit"=T6 252, "marksArray"=w393) -> ("Array"=w399:T5[])  [unwired: 8 in]
          n187 = call "mark_with_max_volume.vi"("marksArray"=w399) -> ("markValue"=w398:T5)
          n188 = Unbundle By Name(w398) -> ("value"=w394:T6)
          n189 = Equal?(x=w397, y=w394) -> (x = y?=w396:bool)
          n190 = Equal To 0?(x=w394) -> (x = 0?=w395:bool)
          n191 = Or(x=w396, y=w395) -> (x .or. y?=w390:bool)
          n192 = case shown="True" w390 {
            tunnel: [w409 w419] -> w405
            tunnel: w391 -> [w410 w418]
            tunnel: [T2 {"type"=enum."empty", "parameter"=0.0} ("action") w417] -> w402
            tunnel: w392 -> [_ w416]
            frame False {
              n193 = Bundle By Name(cluster=w410, "role"=3, "commands"=i32[] []) -> (w409:T11)
            }
            frame True {
              n194 = Unbundle By Name(w418) -> ("commands"=w413:i32[])
              n195 = Delete From Array(array=w413, index=0) -> (deleted portion=w414:i32, array with subset deleted=w412:i32[])  [unwired: 1 in]
              n196 = case shown="121" w414 {
                selector: w414 -> [_ w423 w428 w432 _ _ _]
                tunnel: [T2 {"type"=enum."empty", "parameter"=0.0} ("action") T2 {"type"=enum."empty", "parameter"=0.0} ("action") w427 w431 w436 w442 T2 {"type"=enum."empty", "parameter"=0.0} ("action")] -> w417
                tunnel: w418 -> [w420 w425 w426 w430 w435 w441 w450]
                tunnel: [w420 w424 w426 w430 w435 w441 w451] -> w411
                tunnel: w416 -> [_ _ _ _ _ _ w448]
                frame 0, Default {
                }
                frame 1..8 {
                  n197 = Bundle By Name(cluster=w425, "role"=w423) -> (w424:T11)
                }
                frame 253 {
                  n198 = Bundle By Name(cluster=T2 {"type"=enum."mark", "parameter"=0.0} ("action"), "parameter"=w428) -> (w427:T2)
                }
                frame 255 {
                  n199 = Bundle By Name(cluster=T2 {"type"=enum."mark", "parameter"=0.0} ("action"), "parameter"=w432) -> (w431:T2)
                }
                frame 11 {
                  n200 = Unbundle By Name(w435) -> ("az"=w434:i32)
                  n201 = Bundle By Name(cluster=T2 {"type"=enum."mark", "parameter"=0.0} ("action"), "parameter"=w434) -> (w436:T2)
                }
                frame 12 {
                  n202 = Unbundle By Name(w441) -> ("az"=w440:i32)
                  n203 = Add(x=w440, y=60) -> (x+y=w438:i32)
                  n204 = Bundle By Name(cluster=T2 {"type"=enum."mark", "parameter"=0.0} ("action"), "parameter"=w438) -> (w442:T2)
                }
                frame 121 {
                  n205 = call "current_point_info.vi"("pieceOfWorld"=w448) -> ("marksArray"=w447:T5[])  [unwired: 2 out]
                  n206 = call "range_of_marks.vi"("lower limit"=T6 181, "upper limit"=T6 250, "marksArray"=w447) -> ("Array"=w444:T5[])  [unwired: 8 in]
                  n207 = call "mark_with_max_volume.vi"("marksArray"=w444) -> ("markValue"=w455:T5)
                  n208 = Unbundle By Name(w455) -> ("value"=w454:T6)
                  n209 = Subtract(x=w454, y=183 ("index")) -> (x-y=w453:i32)
                  n210 = Bundle By Name(cluster=w450, "num of az"=w453) -> (w451:T11)
                }
              }
              n211 = Bundle By Name(cluster=w411, "commands"=w412) -> (w419:T11)
            }
          }
          n212 = call "Untitled 2 (SubVI).vi"(11:w405) -> ("appended array"=w403:u32[])  [unwired: 10 in]
        }
        frame 99 {
          n213 = Reshape Array(w459, 9 ("dimension size")) -> (w464:T4[])
          n214 = for {
            tunnel: w464 -> [w467] mode=indexing
            tunnel: [w466] -> w457 mode=concatenating
            n215 = Unbundle By Name(w467) -> ("marksArray"=w466:T5[])
          }
          n216 = call "ant_in_home.vi"("pieceOfWorld"=w459) -> ("x .and. y?"=w460:bool)
          n217 = call "current_point_info.vi"("pieceOfWorld"=w459) -> ("anthillType"=w458:T9, "marksArray"=w456:T5[])  [unwired: 1 out]
          n218 = case shown="False" w460 {
            tunnel: w463 -> [w472 w568]
            tunnel: [w470 w570] -> w461
            tunnel: [w471 w569] -> w462
            tunnel: w458 -> [w473 _]
            tunnel: w457 -> [w469 _]
            tunnel: w456 -> [w468 _]
            frame False {
              n219 = case shown="\"empty\", Default" w473 {
                tunnel: w472 -> [w476 w562]
                tunnel: [w485 w561] -> w471
                tunnel: [w481 w562] -> w470
                tunnel: w469 -> [w475 _]
                tunnel: w468 -> [w474 _]
                frame "empty", Default {
                  n220 = Index Array(array=w476, index=1) -> (element=w478:u8)
                  n221 = Add(x=w478, y=u8 2) -> (x+y=w483:u8)
                  n222 = Quotient & Remainder(x=w483, y=u8 4) -> (x-y*floor(x/y)=w480:u8)  [unwired: 1 out]
                  n223 = call "mark_volume.vi"("element"=w480, "marksArray"=w475) -> ("volume"=w479:T7)  [unwired: 9 in]
                  n224 = call "mark_volume.vi"("element"=w478, "marksArray"=w475) -> ("volume"=w477:T7)  [unwired: 9 in]
                  n225 = case shown="Default" w479 {
                    tunnel: [w488 w522] -> w485
                    tunnel: w476 -> [w490 w523]
                    tunnel: [w489 w524] -> w481
                    tunnel: w477 -> [w491 w521]
                    tunnel: w474 -> [w487 w520]
                    frame 0 {
                      n226 = case shown="Default" w491 {
                        tunnel: w490 -> [w494 w505]
                        tunnel: [w494 w505] -> w489
                        tunnel: [w493 w511] -> w488
                        tunnel: w487 -> [_ w509]
                        frame 0 {
                          n227 = Index Array(array=w494, index=1) -> (element=w495:u8)
                          n228 = Bundle By Name(cluster=T2 {"type"=enum."mark", "parameter"=0.0} ("action"), "parameter"=w495) -> (w493:T2)
                        }
                        frame Default {
                          n229 = Index Array(array=w505, index=1) -> (element=w508:u8)
                          n230 = Array Subset(array=w505, index=3, length=2) -> (w504:u8[])
                          n231 = call "mark_volume.vi"("element"=w508, "marksArray"=w509) -> ("volume"=w503:T7)  [unwired: 9 in]
                          n232 = call "256_to_10.vi"("Array"=w504) -> ("Numeric"=w499:dbl)
                          n233 = Subtract(x=w499, y=1.0) -> (x-y=w497:dbl)
                          n234 = Less?(x=w503, y=w497) -> (x < y?=w501:bool)
                          n235 = Greater Than 0?(x=w503) -> (x > 0?=w502:bool)
                          n236 = And(x=w502, y=w501) -> (x .and. y?=w500:bool)
                          n237 = case shown="True" w500 {
                            tunnel: [w514 w517] -> w511
                            tunnel: w508 -> [w512 w518]
                            frame False {
                              n238 = Multiply(x=w512, y=1.5707963267948966) -> (x*y=w515:dbl)
                              n239 = Bundle By Name(cluster=T2 {"type"=enum."move", "parameter"=0.0} ("action"), "parameter"=w515) -> (w514:T2)
                            }
                            frame True {
                              n240 = Bundle By Name(cluster=T2 {"type"=enum."mark", "parameter"=0.0} ("action"), "parameter"=w518) -> (w517:T2)
                            }
                          }
                        }
                      }
                    }
                    frame Default {
                      n241 = case shown="Default" w521 {
                        tunnel: [w538 w557] -> w524
                        tunnel: w523 -> [w529 w557]
                        tunnel: [w539 w559] -> w522
                        tunnel: w520 -> [w530 _]
                        frame Default {
                          n242 = Index Array(array=w529, index=1) -> (element=w527:u8)
                          n243 = Array Subset(array=w529, index=3, length=2) -> (w534:u8[])
                          n244 = call "mark_volume.vi"("element"=w527, "marksArray"=w530) -> ("volume"=w533:T7)  [unwired: 9 in]
                          n245 = call "256_to_10.vi"("Array"=w534) -> ("Numeric"=w526:dbl)
                          n246 = Decrement(x=w526) -> (x-1=w525:dbl)
                          n247 = Greater Than 0?(x=w533) -> (x > 0?=w532:bool)
                          n248 = Less?(x=w533, y=w525) -> (x < y?=w531:bool)
                          n249 = And(x=w531, y=w532) -> (x .and. y?=w528:bool)
                          n250 = case shown="False" w528 {
                            tunnel: [w550 w552] -> w539
                            tunnel: w529 -> [w542 w555]
                            tunnel: [w541 w555] -> w538
                            tunnel: w527 -> [_ w553]
                            frame False {
                              n251 = Index Array(array=w542, index=1) -> (element=w545:u8)
                              n252 = Increment(x=w545) -> (x+1=w547:u8)
                              n253 = Quotient & Remainder(x=w547, y=u8 4) -> (x-y*floor(x/y)=w540:u8)  [unwired: 1 out]
                              n254 = Multiply(x=w540, y=1.5707963267948966) -> (x*y=w548:dbl)
                              n255 = Replace Array Subset(array=w542, new element=w540, index=1) -> (w541:u8[])
                              n256 = Bundle By Name(cluster=T2 {"type"=enum."move", "parameter"=0.0} ("action"), "parameter"=w548) -> (w550:T2)
                            }
                            frame True {
                              n257 = Bundle By Name(cluster=T2 {"type"=enum."mark", "parameter"=0.0} ("action"), "parameter"=w553) -> (w552:T2)
                            }
                          }
                        }
                        frame 0 {
                          n258 = Index Array(array=w557, index=1) -> (element=w558:u8)
                          n259 = Bundle By Name(cluster=T2 {"type"=enum."mark", "parameter"=0.0} ("action"), "parameter"=w558) -> (w559:T2)
                        }
                      }
                    }
                  }
                }
                frame "own" {
                  n260 = Index Array(array=w562, index=1) -> (element=w564:u8)
                  n261 = Multiply(x=w564, y=1.5707963267948966) -> (x*y=w566:dbl)
                  n262 = Bundle By Name(cluster=T2 {"type"=enum."move", "parameter"=0.0} ("action"), "parameter"=w566) -> (w561:T2)
                }
              }
            }
            frame True {
              n263 = Index Array(array=w568, index=2) -> (element=w576:u8)
              n264 = Replace Array Subset(array=w568, new element=w576, index=1) -> (w570:u8[])
              n265 = Index Array(array=w570, index=1) -> (element=w572:u8)
              n266 = Multiply(x=w572, y=1.5707963267948966) -> (x*y=w574:dbl)
              n267 = Bundle By Name(cluster=T2 {"type"=enum."move", "parameter"=0.0} ("action"), "parameter"=w574) -> (w569:T2)
            }
          }
        }
        frame 180 {
          # "Administrator"
          n268 = call "array_to_memo_admin.vi"("memory"=w583) -> (3:w581:T10)  [unwired: 10 in]
          n269 = Unbundle By Name(w581) -> ("vol step"=w582:i32)
          n270 = call "current_point_info.vi"("pieceOfWorld"=w585) -> ("marksArray"=w584:T5[])  [unwired: 2 out]
          n271 = case shown="Default" w582 {
            selector: w582 -> [_ w611]
            tunnel: [w590 w618] -> w586
            tunnel: [w587 w617] -> w580
            tunnel: w584 -> [w591 w616]
            tunnel: w581 -> [w588 w609]
            frame 0 {
              n272 = Unbundle By Name(w588) -> ("max vol"=w589:i32)
              n273 = call "mark_volume.vi"("element"=T6 182, "marksArray"=w591) -> ("volume"=w592:T7)  [unwired: 9 in]
              n274 = Subtract(x=w589, y=w592) -> (x-y=w594:i32)
              n275 = case shown="Default" w594 {
                selector: w594 -> [_ w599]
                tunnel: [w595 w597] -> w587
                tunnel: w591 -> [_ w605]
                tunnel: [T2 {"type"=enum."empty", "parameter"=0.0} ("action") T2 {"type"=enum."mark", "parameter"=251.0} ("action")] -> w590
                tunnel: w588 -> [w595 w600]
                frame 0 {
                }
                frame Default {
                  n276 = call "range_of_marks.vi"("lower limit"=T6 181, "upper limit"=T6 250, "marksArray"=w605) -> ("Array"=w602:T5[])  [unwired: 8 in]
                  n277 = call "mark_with_max_volume.vi"("marksArray"=w602) -> ("markValue"=w607:T5)
                  n278 = Unbundle By Name(w607) -> ("value"=w606:T6)
                  n279 = Subtract(x=w606, y=183 ("index")) -> (x-y=w598:i32)
                  n280 = Bundle By Name(cluster=w600, "vol step"=w599, "num of az"=w598) -> (w597:T10)
                }
              }
            }
            frame Default {
              n281 = Unbundle By Name(w609) -> ("max vol"=w610:i32)
              n282 = call "mark_volume.vi"("element"=T6 253, "marksArray"=w616) -> ("volume"=w612:T7)  [unwired: 9 in]
              n283 = Subtract(x=w610, y=w612) -> (x-y=w614:i32)
              n284 = Less Or Equal?(x=w614, y=w611) -> (x <= y?=w613:bool)
              n285 = case shown="True" w613 {
                tunnel: [w623 w659] -> w618
                tunnel: w609 -> [w619 w653]
                tunnel: [w619 w654] -> w617
                tunnel: w616 -> [w621 w660]
                tunnel: w612 -> [_ w658]
                tunnel: w611 -> [_ w657]
                frame False {
                  n286 = call "mark_volume.vi"("element"=T6 181, "marksArray"=w621) -> ("volume"=w622:T7)  [unwired: 9 in]
                  n287 = case shown="Default" w622 {
                    tunnel: [w629 T2 {"type"=enum."mark", "parameter"=181.0} ("action")] -> w623
                    tunnel: w619 -> [w626 _]
                    tunnel: w621 -> [w628 _]
                    frame Default {
                      n288 = Unbundle By Name(w626) -> ("arr of az"=w625:i32[], "mode mark"=w624:i32)
                      n289 = call "mark_volume.vi"("element"=w624, "marksArray"=w628) -> ("volume"=w627:T7)  [unwired: 9 in]
                      n290 = case shown="Default" w627 {
                        tunnel: [w631 w636] -> w629
                        tunnel: w628 -> [_ w635]
                        tunnel: w625 -> [_ w634]
                        tunnel: w624 -> [w630 _]
                        frame 0..1000 {
                          n291 = Bundle By Name(cluster=T2 {"type"=enum."mark", "parameter"=0.0} ("action"), "parameter"=w630) -> (w631:T2)
                        }
                        frame Default {
                          n292 = Array Size(array=w634) -> (size(s)=w633:i32)
                          n293 = case shown="Default" w633 {
                            tunnel: [T2 {"type"=enum."empty", "parameter"=0.0} ("action") w644] -> w636
                            tunnel: w635 -> [_ w643]
                            tunnel: w634 -> [_ w639]
                            frame 0 {
                            }
                            frame Default {
                              n294 = Index Array(array=w639) -> (element=w638:i32)  [unwired: 1 in]
                              n295 = Add(x=w638, y=u8 120) -> (x+y=w641:i32)
                              n296 = call "mark_volume.vi"("element"=w641, "marksArray"=w643) -> ("volume"=w640:T7)  [unwired: 9 in]
                              n297 = case shown="0..1000" w640 {
                                tunnel: [T2 {"type"=enum."empty", "parameter"=0.0} ("action") w648] -> w644
                                tunnel: w641 -> [_ w647]
                                frame Default {
                                }
                                frame 0..1000 {
                                n298 = Bundle By Name(cluster=T2 {"type"=enum."mark", "parameter"=0.0} ("action"), "parameter"=w647) -> (w648:T2)
                                }
                              }
                            }
                          }
                        }
                      }
                    }
                    frame 0..1000 {
                    }
                  }
                }
                frame True {
                  n299 = for {
                    tunnel: w660 -> [w686] mode=indexing
                    shift-right: [w684] -> w650
                    shift-left: w653 -> [w685]
                    tunnel: w658 -> [w680]
                    tunnel: w657 -> [w677]
                    n300 = Unbundle By Name(w686) -> ("volume"=w679:T7, "value"=w683:T6)
                    n301 = Multiply(x=2 ("y"), y=w677) -> (x*y=w676:i32)
                    n302 = Subtract(x=w680, y=w679) -> (x-y=w682:T7)
                    n303 = Less Or Equal?(x=w682, y=w676) -> (x <= y?=w681:bool)
                    n304 = case shown="True" w681 {
                      tunnel: w685 -> [w687 w688]
                      tunnel: [w687 w689] -> w684
                      tunnel: w683 -> [_ w690]
                      frame False {
                      }
                      frame True {
                        n305 = in-place {
                          in-place-border: w690 -> [w695]
                          n306 = in-place-cluster #4(w688) -> ("arr of blk"=w694:i32[], "arr of az"=w692:i32[])
                          n307 = case shown="1..60" w695 {
                            selector: w695 -> [_ w702 w714]
                            tunnel: w694 -> [w697 w700 w710]
                            tunnel: [w697 w700 w709] -> w693
                            tunnel: w692 -> [w696 w699 w708]
                            tunnel: [w696 w698 w707] -> w691
                            frame Default {
                            }
                            frame 1..60 {
                              n308 = Search 1D Array(1D array=w699, element=w702) -> (index of element=w701:i32)  [unwired: 1 in]
                              n309 = case shown="-1" w701 {
                                tunnel: w699 -> [w703 w706]
                                tunnel: [w703 w705] -> w698
                                tunnel: w702 -> [_ w704]
                                frame Default {
                                }
                                frame -1 {
                                n310 = Insert Into Array(array=w706, new element=w704) -> (w705:i32[])  [unwired: 1 in]
                                }
                              }
                            }
                            frame 61..120 {
                              n311 = Subtract(x=w714, y=T6 60) -> (x-y=w712:T6)
                              n312 = Search 1D Array(1D array=w708, element=w712) -> (index of element=w716:i32)  [unwired: 1 in]
                              n313 = Decrement(x=w712) -> (x-1=w711:T6)
                              n314 = case shown="Default" w716 {
                                selector: w716 -> [_ w719]
                                tunnel: w708 -> [w717 w720]
                                tunnel: [w717 w718] -> w707
                                frame -1 {
                                }
                                frame Default {
                                n315 = Delete From Array(array=w720, index=w719) -> (array with subset deleted=w718:i32[])  [unwired: 1 in, 1 out]
                                }
                              }
                              n316 = Replace Array Subset(array=w710, new element=u8 1 ("new element/subarray"), index=w711) -> (w709:i32[])
                            }
                          }
                          n317 = in-place-cluster #4("arr of blk"=w693, "arr of az"=w691) -> (w689:T10)
                        }
                      }
                    }
                  }
                  n318 = Unbundle By Name(w650) -> ("arr of blk"=w652:i32[], "num of az"=w651:i32)
                  n319 = Add Array Elements(numeric array=w652) -> (sum=w656:i32)
                  n320 = Equal?(x=w656, y=w651) -> (x = y?=w655:bool)
                  n321 = case shown="False" w655 {
                    tunnel: [T2 {"type"=enum."empty", "parameter"=0.0} ("action") w666] -> w659
                    tunnel: w650 -> [w662 w663]
                    tunnel: [w662 w664] -> w654
                    frame False {
                    }
                    frame True {
                      n322 = in-place {
                        in-place-border: [w669] -> w665
                        n323 = in-place-cluster #5(w663) -> ("mode mark"=w671:i32)  [unwired: 2 out]
                        n324 = case shown="252" w671 {
                          tunnel: [252 251] -> w669
                          frame 251, Default {
                          }
                          frame 252 {
                          }
                        }
                        n325 = Initialize Array(0, 60 ("dimension size")) -> (w668:i32[])
                        n326 = in-place-cluster #5("role"=181, "mode mark"=w669, "arr of blk"=w668) -> (w664:T10)
                      }
                      n327 = Bundle By Name(cluster=T2 {"type"=enum."mark", "parameter"=0.0} ("action"), "parameter"=w665) -> (w666:T2)
                    }
                  }
                }
              }
            }
          }
          n328 = call "memo_ta_array_admin.vi"("Cluster"=w580) -> ("appended array"=w579:u32[])  [unwired: 10 in]
        }
        frame 181 {
          n329 = Replace Array Subset(array=w723, new element=u8 182 ("new element/subarray"), index=0) -> (w722:u8[])
        }
        frame 182 {
          n330 = Replace Array Subset(array=w728, new element=u8 180 ("new element/subarray"), index=0) -> (w727:u8[])
        }
      }
    }
    frame True {
      # "Ant's memory is empty"
      n331 = call "current_point_info.vi"("pieceOfWorld"=w732) -> ("marksArray"=w731:T5[])  [unwired: 2 out]
      n332 = Empty Array?(array=w731) -> (empty?=w735:bool)
      n333 = case shown="False" w735 {
        tunnel: [w743 w813] -> w736
        tunnel: [w742 w810] -> w734
        tunnel: w733 -> [_ _]
        tunnel: w731 -> [w741 _]
        frame False {
          n334 = call "mark_with_max_volume.vi"("marksArray"=w741) -> ("markValue"=w740:T5)
          n335 = Unbundle By Name(w740) -> ("volume"=w738:T7, "value"=w739:T6)
          n336 = case shown="181" w739 {
            selector: w739 -> [w757 w771 w786 w797]
            tunnel: [w755 w773 w790 w800] -> w743
            tunnel: [w749 w772 w789 w798] -> w742
            tunnel: w738 -> [w756 w766 _ _]
            frame 181 {
              w751 = T6 0 ("element")
              n337 = call "10_to_256.vi"("Decimal"=w756) -> ("256"=w760:u8[])
              n338 = Index Array(array=w760) -> (element #1=w753:u8, element #2=w754:u8, element #3=w752:u8)  [unwired: 3 in]
              n339 = Increment(x=w757) -> (x+1=w758:T6)
              n340 = Build Array(T6 180 ("element"), w753, w754, w752, w751, w751, T6 0 ("element"), T6 251 ("element")) -> (w750:T6[])
              n341 = Initialize Array(T6 0 ("element"), 60 ("dimension size")) -> (w746:T6[])
              n342 = Insert Into Array(array=w750, new element=w746) -> (w749:T6[])  [unwired: 1 in]
              n343 = Bundle By Name(cluster=T2 {"type"=enum."mark", "parameter"=0.0} ("action"), "parameter"=w758) -> (w755:T2)
            }
            frame 182, 183 {
              w765 = T6 0 ("element")
              n344 = call "10_to_256.vi"("Decimal"=w766) -> ("256"=w764:u8[])
              n345 = Subtract(x=w771, y=T6 182) -> (x-y=w770:T6)
              n346 = Increment(x=w771) -> (x+1=w776:T6)
              n347 = Index Array(array=w764) -> (element #1=w763:u8, element #2=w762:u8)  [unwired: 2 in]
              n348 = Multiply(x=w770, y=T6 2) -> (x*y=w768:T6)
              n349 = Build Array(T6 9 ("element"), w768, w768, w763, w762, w765, w765, w765, w765, w765, w765, w765, w765, w765, T6 0 ("element")) -> (w772:T6[])
              n350 = Bundle By Name(cluster=T2 {"type"=enum."mark", "parameter"=0.0} ("action"), "parameter"=w776) -> (w773:T2)
            }
            frame 184..242 {
              w785 = T6 0 ("element")
              # "Ant became a ranger"
              n351 = Increment(x=w786) -> (x+1=w788:T6)
              n352 = Subtract(x=w786, y=T6 182) -> (x-y=w783:T6)
              n353 = Build Array(T6 8 ("element"), w783, w785, w785, w785, w785, w785, w785, w785, w785, T6 251 ("element"), w783, w785, w785, T6 0 ("element"), T6 121 ("element"), T6 1 ("element"), T6 0 ("element")) -> (w789:T6[])
              n354 = Bundle By Name(cluster=T2 {"type"=enum."mark", "parameter"=0.0} ("action"), "parameter"=w788) -> (w790:T2)
            }
            frame Default {
              w795 = T6 0 ("element")
              # "Ant became an ant-on-duty"
              n355 = Build Array(T6 3 ("element"), w795, w795, w795, w795, w795, w795, w795, w795, w795, T6 251 ("element"), T6 0 ("element"), T6 60 ("element"), w795, T6 0 ("element")) -> (w798:T6[])
              n356 = Bundle By Name(cluster=T2 {"type"=enum."mark", "parameter"=0.0} ("action"), "parameter"=w797) -> (w800:T2)
            }
          }
        }
        frame True {
          w806 = T6 0 ("element")
          w807 = T6 1 ("element")
          # "The very first ant"
          n357 = Bundle By Name(cluster=T2 {"type"=enum."mark", "parameter"=0.0} ("action"), "parameter"=T6 181 ("element")) -> (w813:T2)
          n358 = Build Array(T6 8 ("element"), w807, w806, w806, w806, w806, w806, w806, w806, w806, T6 251 ("element"), w807, w806, w806, T6 0 ("element"), T6 121 ("element"), T6 1 ("element"), T6 0 ("element")) -> (w810:T6[])
        }
      }
    }
  }
  "error out" <- w5
  "action" <- w13
  n359 = call "memory_set.vi"("memory"=w7, "ant_base in"=w8) -> ("ant_base out"=→"Igor out":refnum<class "PolyVIEW.lvclass">)  [unwired: 8 in, 1 out]
